vi "Config 135 via GPIB.vi"(3 "error in":T1, 4 "Configuration (in)":T3={"Sensor Length (cm)"=100.0, "Hi Setpoint (cm)"=80.0, "Lo Setpoint (cm)"=20.0, "Sampling Interval (min)"=1.0} {"Sampling Interval (min)" min=0 max=600 format="%.1f"; "Lo Setpoint (cm)" min=0 max=203.2 format="%.1f"; "Hi Setpoint (cm)" min=0 max=203.2 format="%.1f"; "Sensor Length (cm)" min=1 max=203.2 format="%.1f"}, 5 "Hidden Controls (in)":T2 {"Prev Sampling Interval" format="%.1f"; "Prev Lo Setpoint" format="%.1f"; "Prev Hi Setpoint" format="%.1f"; "Prev Sensor Length" format="%.1f"; "Helium Level (cm)" format="%.1f"}, 6 "GPIB Setup":cluster{"GPIB address":i16, "GPIB bus":i16}={"GPIB address"=1, "GPIB bus"=0}) -> (0 "error out":T1, 1 "Hidden Controls (out)":T2 {"Prev Sampling Interval" format="%.1f"; "Prev Lo Setpoint" format="%.1f"; "Prev Hi Setpoint" format="%.1f"; "Prev Sensor Length" format="%.1f"; "Helium Level (cm)" format="%.1f"}, 2 "Configuration (out)":T3={"Sensor Length (cm)"=100.0, "Hi Setpoint (cm)"=80.0, "Lo Setpoint (cm)"=20.0, "Sampling Interval (min)"=1.0} {"Sampling Interval (min)" min=0 max=600 format="%.1f"; "Lo Setpoint (cm)" min=0 max=203.2 format="%.1f"; "Hi Setpoint (cm)" min=0 max=203.2 format="%.1f"; "Sensor Length (cm)" min=1 max=203.2 format="%.1f"})   [LabVIEW 2019]
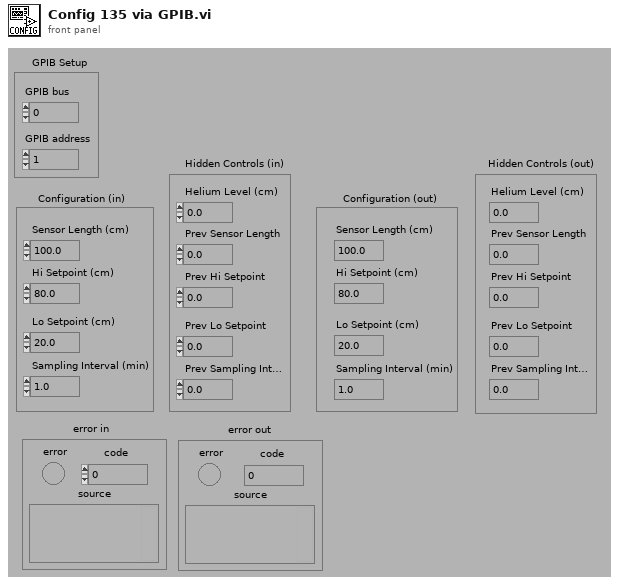
[diagram p1: front panel]
types:
  T1 = cluster{"error":bool, "code":i32, "source":string}
  T2 = cluster{"Helium Level (cm)":sgl, "Prev Sensor Length":sgl, "Prev Hi Setpoint":sgl, "Prev Lo Setpoint":sgl, "Prev Sampling Interval":sgl}
  T3 = cluster{"Sensor Length (cm)":sgl, "Hi Setpoint (cm)":sgl, "Lo Setpoint (cm)":sgl, "Sampling Interval (min)":sgl}
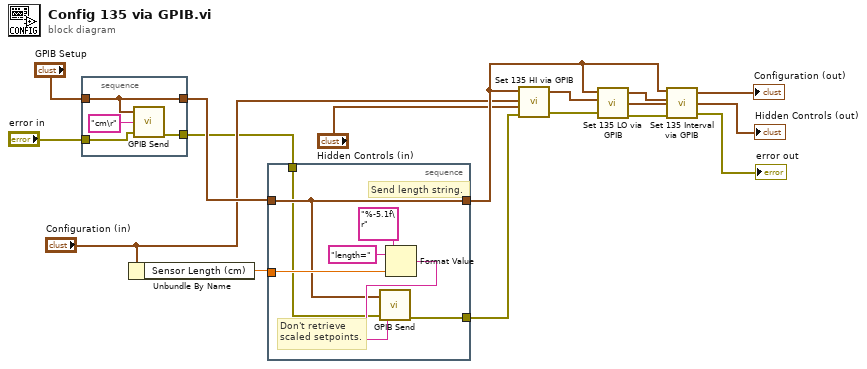
[diagram p0: block diagram]
diagram:
  n1 = stacked-sequence {
    tunnel: "GPIB Setup" -> [w21]
    tunnel: [w21] -> w16
    tunnel: [w20] -> w7
    tunnel: "error in" -> [w18]
    frame #0 {
      n2 = call "GPIB Send.vi"("GPIB Setup"=w21, "Input command"="cm\r", "error in"=w18) -> ("error out"=w20:T1)  [unwired: 3 out]
    }
  }
  n3 = Unbundle By Name("Configuration (in)") -> ("Sensor Length (cm)"=w15:sgl)
  n4 = stacked-sequence {
    tunnel: w15 -> [w27]
    tunnel: w16 -> [w24]
    tunnel: [w24] -> w14
    tunnel: w7 -> [w23]
    tunnel: [w22] -> w6
    frame #0 {
      # "Don't retrieve\nscaled setpoints."
      # "Send length string."
      n5 = Format Value(string ("")="length=", format string="%-5.1f\r", value (0)=w27) -> (output string=w28:string)
      n6 = call "GPIB Send.vi"("GPIB Setup"=w24, "Input command"=w28, "error in"=w23) -> ("error out"=w22:T1)  [unwired: 3 out]
    }
  }
  n7 = call "Set 135 HI via GPIB.vi"("error in"=w6, "Hidden Controls (in)"="Hidden Controls (in)", "Configuration (in)"="Configuration (in)", "GPIB Setup"=w14) -> ("error out"=w9:T1, "Configuration (out)"=w3:T3)  [unwired: 1 out]
  n8 = call "Set 135 LO via GPIB.vi"("error in"=w9, "Configuration (in)"=w3, "GPIB Setup"=w14) -> ("error out"=w8:T1, "Hidden Controls (out)"=w1:T2, "Configuration (out)"=w2:T3)  [unwired: 1 in]
  n9 = call "Set 135 Interval via GPIB.vi"("error in"=w8, "Hidden Controls (in)"=w1, "Configuration (in)"=w2, "GPIB Setup"=w14) -> ("error out"=→"error out":T1, "Hidden Controls (out)"=→"Hidden Controls (out)":T2, "Configuration (out)"=→"Configuration (out)":T3)
